vi "READ.vi"(8 "error in (no error)":errorcluster, 10 "unsigned byte array 2":u8[](array[numeric]), 11 "VISA resource name":refnum<visa-resource-name>) -> (0 "error out":errorcluster, 2 "unsigned byte array":u8[](array[numeric]), 3 "VISA resource name out":refnum<visa-resource-name>)   [LabVIEW 2018]
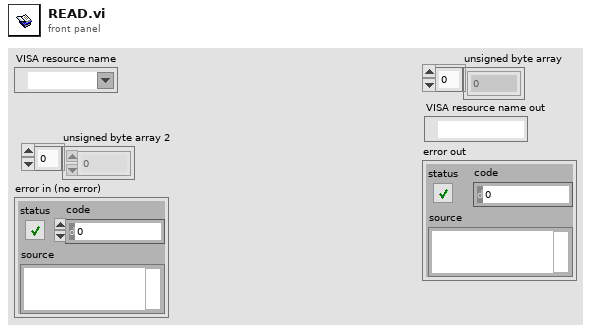
[diagram p1: front panel]
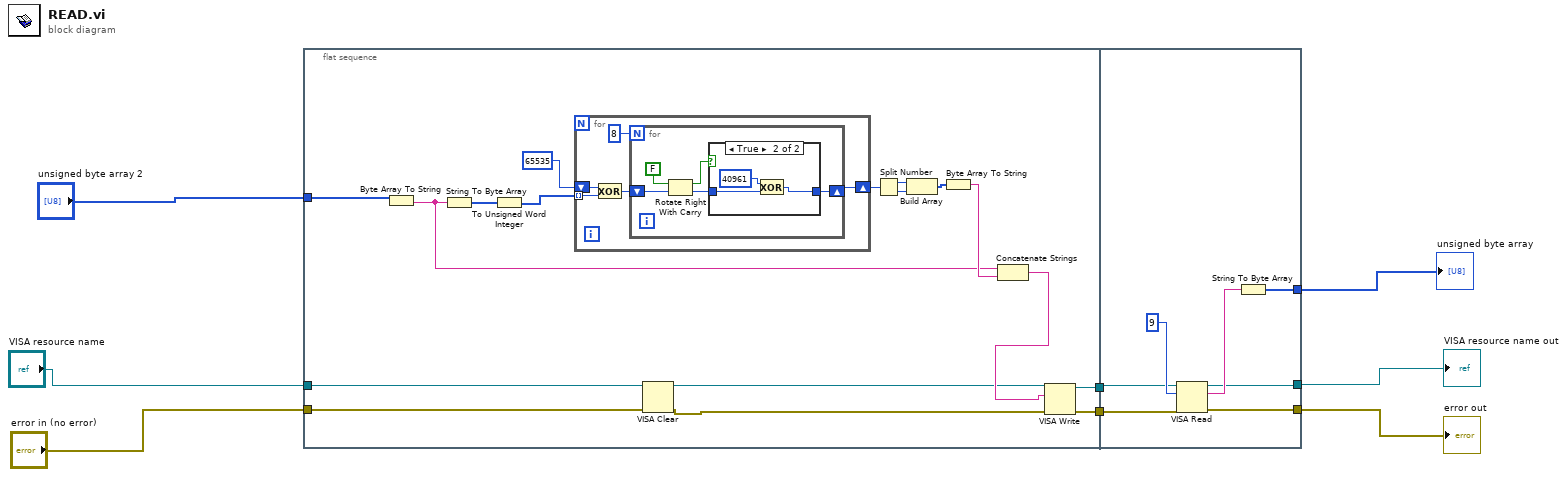
[diagram p0: block diagram]
diagram:
  n1 = flat-sequence {
    tunnel: [w13] -> w8
    tunnel: [w12] -> w7
    tunnel: "unsigned byte array 2" -> [w11]
    tunnel: "error in (no error)" -> [w10]
    tunnel: "VISA resource name" -> [w9]
    tunnel: w8 -> [w44]
    tunnel: w7 -> [w43]
    tunnel: [w42] -> w6
    tunnel: [w41] -> w5
    tunnel: [w40] -> w4
    frame #0 {
      n2 = Byte Array To String(unsigned byte array=w11) -> (string=w19:string)
      n3 = String To Byte Array(string=w19) -> (unsigned byte array=w23:u8[])
      n4 = To Unsigned Word Integer(number=w23) -> (unsigned 16bit integer=w24:u16[])
      n5 = for {
        shift-right: [w27] -> w25
        shift-left: u16 65535 -> [w28]
        tunnel: w24 -> [w26] mode=indexing
        n6 = Exclusive Or(1:w26, 2:w28) -> (0:w29:u16)
        n7 = for {
          N: 8 -> [_]
          shift-right: [w34] -> w27
          shift-left: w29 -> [w33]
          n8 = Rotate Right With Carry(2:w33, 3:FALSE ("Übertrag")) -> (0:w35:u16, 1:w32:bool)
          n9 = case shown="True" w32 {
            tunnel: w35 -> [w36 w38]
            tunnel: [w36 w37] -> w34
            frame False {
            }
            frame True {
              n10 = Exclusive Or(1:w38, 2:u16 40961) -> (0:w37:u16)
            }
          }
        }
      }
      n11 = VISA Clear(VISA resource name=w9, error in (no error)=w10) -> (VISA resource name out=w14:refnum<visa-resource-name>, error out=w15:errorcluster)
      n12 = Split Number(x=w25) -> (hi(x)=w22:u8, lo(x)=w21:u8)
      n13 = Build Array(w22, w21) -> (w18:u8[])
      n14 = Byte Array To String(unsigned byte array=w18) -> (string=w20:string)
      n15 = Concatenate Strings(w19, w20) -> (w16:string)
      n16 = VISA Write(VISA resource name=w14, write buffer=w16, error in (no error)=w15) -> (VISA resource name out=w13:refnum<visa-resource-name>, error out=w12:errorcluster)  [unwired: 1 out]
    }
    frame #1 {
      n17 = VISA Read(VISA resource name=w44, byte count=u32 9, error in (no error)=w43) -> (VISA resource name out=w41:refnum<visa-resource-name>, read buffer=w45:string, error out=w40:errorcluster)  [unwired: 1 out]
      n18 = String To Byte Array(string=w45) -> (unsigned byte array=w42:u8[])
    }
  }
  "unsigned byte array" <- w6
  "VISA resource name out" <- w5
  "error out" <- w4
